vi "TalonFXCommandPosition.vi"(0 "Device Reference (in)":T2, 5 "Output Mode":T1(ring), 7 "Control Mode":enum16{"Safety", "Travelling", "Positioning"}(ring), 9 "Position (counts) or Testing Power":dbl, 11 "Error (in)":errorcluster, 12 "Feed Forward Power [-1, 1]":dbl) -> ()   [LabVIEW 2020]
doc: "Wrapper for commanding the postion of a Talon SRX motor controller. Supports PID, Motion Magic, and a safety interlock. Also supports the standard actuator testing interface and and the only sending new values on change."
uses:
  <vilib>/Rock Robotics/WPI/MotorControl/WPI_MotorControlDeviceRef.ctl
  <vilib>/Rock Robotics/WPI/MotorControl/WPI_MotorControlType.ctl
  <vilib>/Rock Robotics/SystemInterfaces/DIO/FPGA_DIOPWMChannel.ctl
  <vilib>/Rock Robotics/WPI/PWM/WPI_PWMDeadband.ctl
  <vilib>/Rock Robotics/SystemInterfaces/DIO/FPGA_DIOChannel.ctl
  <vilib>/Rock Robotics/WPI/ThirdParty/Phoenix-LabVIEW/Motor Controller/Controls/CTRE_Phoenix_MotorControl_ControlMode.ctl
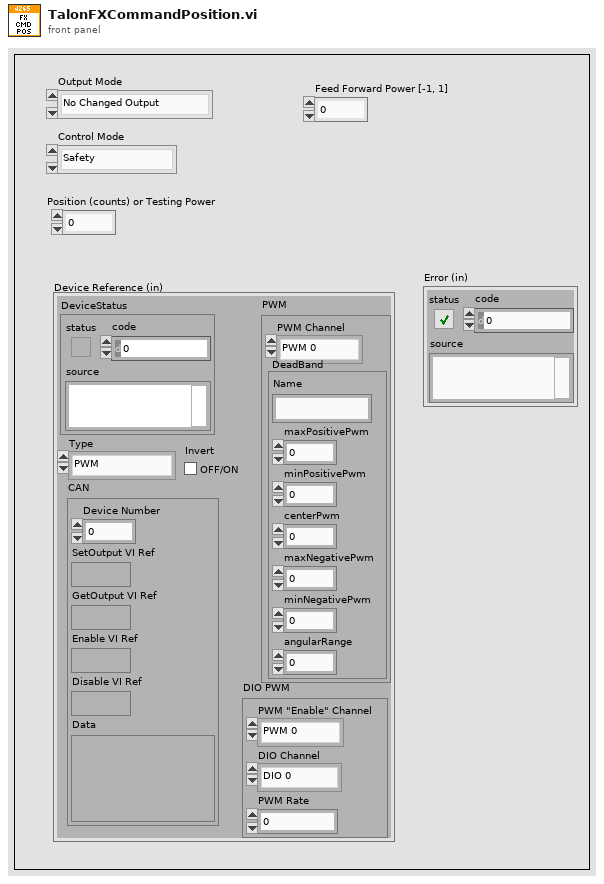
[diagram p1: front panel]
types:
  T1 = enum16{"No Changed Output", "New Normal Output", "New Testing Output"}
  T2 = typedef "WPI_MotorControlDeviceRef.ctl" = cluster{"DeviceStatus":errorcluster, "Type":T3, "PWM":cluster{"PWM Channel":T4, "DeadBand":T5}, "CAN":cluster{"Device Number":u8, "SetOutput VI Ref":variant, "GetOutput VI Ref":variant, "Enable VI Ref":variant, "Disable VI Ref":variant, "Data":variant}, "Invert":bool, "DIO PWM":cluster{"PWM \"Enable\" Channel":T4, "DIOChannel":T6, "PWM Rate":dbl}}
  T3 = typedef "WPI_MotorControlType.ctl" = enum16{"PWM", "CAN", "DIO PWM"}
  T4 = typedef "FPGA_DIOPWMChannel.ctl" = enum8{"PWM 0", "PWM 1", "PWM 2", "PWM 3", "PWM 4", "PWM 5", "PWM 6", "PWM 7", "PWM 8", "PWM 9", "PWM MXP 0", "PWM MXP 1", "PWM MXP 2", "PWM MXP 3", "PWM MXP 4", "PWM MXP 5", "PWM MXP 6", "PWM MXP 7", "PWM MXP 8", "PWM MXP 9", "Invalid"}
  T5 = typedef "WPI_PWMDeadband.ctl" = cluster{"Name":string, "maxPositivePwm":i32, "minPositivePwm":i32, "centerPwm":i32, "maxNegativePwm":i32, "minNegativePwm":i32, "angularRange":u16}
  T6 = typedef "FPGA_DIOChannel.ctl" = enum8{"DIO 0", "DIO 1", "DIO 2", "DIO 3", "DIO 4", "DIO 5", "DIO 6", "DIO 7", "DIO 8", "DIO 9", "DIO MXP 0", "DIO MXP 1", "DIO MXP 2", "DIO MXP 3", "DIO MXP 4", "DIO MXP 5", "DIO MXP 6", "DIO MXP 7", "DIO MXP 8", "DIO MXP 9", "DIO MXP 10", "DIO MXP 11", "DIO MXP 12", "DIO MXP 13", "DIO MXP 14", "DIO MXP 15", "SPI Port CS1", "SPI Port CS2", "SPI Port CS3", "SPI Port MISO", "SPI Port MOSI", "Invalid"}
  T7 = enum16{"DemandType_Neutral", "DemandType_AuxPID", "DemandType_ArbitraryFeedForward"}
  T8 = typedef "CTRE_Phoenix_MotorControl_ControlMode.ctl" = u16
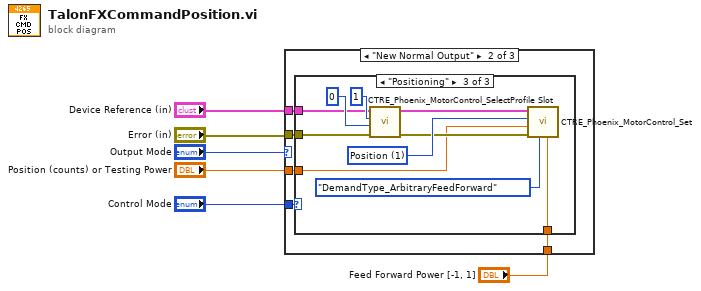
[diagram p0: block diagram]
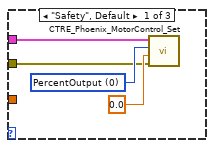
[diagram p3: hidden frame]
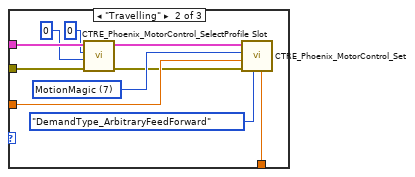
[diagram p4: hidden frame]
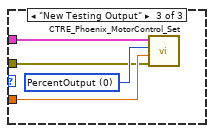
[diagram p5: hidden frame]
diagram:
  n1 = case shown="\"New Normal Output\"" "Output Mode" {
    tunnel: "Position (counts) or Testing Power" -> [_ w10 w38]
    tunnel: "Device Reference (in)" -> [_ w9 w39]
    tunnel: "Feed Forward Power [-1, 1]" -> [_ w11 _]
    tunnel: "Control Mode" -> [_ w8 _]
    tunnel: "Error (in)" -> [_ w7 w36]
    frame "No Changed Output", Default {
    }
    frame "New Normal Output" {
      n2 = case shown="\"Positioning\"" w8 {
        tunnel: w9 -> [w15 w21 w29]
        tunnel: w10 -> [_ w24 w27]
        tunnel: w11 -> [_ w22 w26]
        tunnel: w7 -> [w12 w16 w28]
        frame "Safety", Default {
          w14 = T8 0 items=["PercentOutput"=0, "Position"=1, "Velocity"=2, "Current"=3, "Follower"=5, "MotionProfile"=6, "MotionMagic"=7, "MotionProfileArc"=10, "Disabled"=15] ("Control Mode")
          n3 = call <vilib>:"CTRE_Phoenix_MotorControl_Set.vi"("error in (no error)"=w12, "Output"=0.0, "Control Mode"=w14, "PhoenixMotorControlDevRef"=w15) -> ()  [unwired: 6 in, 2 out]
        }
        frame "Travelling" {
          w25 = T8 7 items=["PercentOutput"=0, "Position"=1, "Velocity"=2, "Current"=3, "Follower"=5, "MotionProfile"=6, "MotionMagic"=7, "MotionProfileArc"=10, "Disabled"=15] ("Control Mode")
          n4 = call <vilib>:"CTRE_Phoenix_MotorControl_SelectProfile Slot.vi"("error in (no error)"=w16, "pidLoopIdx"=0, "slotIdx"=0, "PhoenixMotorControlDevRef"=w21) -> ("error out"=w17:errorcluster, "PhoenixMotorControlDevRef"=w20:T2)  [unwired: 6 in]
          n5 = call <vilib>:"CTRE_Phoenix_MotorControl_Set.vi"("Demand1"=w22, "DemandType"=T7."DemandType_ArbitraryFeedForward", "error in (no error)"=w17, "Output"=w24, "Control Mode"=w25, "PhoenixMotorControlDevRef"=w20) -> ()  [unwired: 4 in, 2 out]
        }
        frame "Positioning" {
          w35 = T8 1 items=["PercentOutput"=0, "Position"=1, "Velocity"=2, "Current"=3, "Follower"=5, "MotionProfile"=6, "MotionMagic"=7, "MotionProfileArc"=10, "Disabled"=15] ("Control Mode")
          n6 = call <vilib>:"CTRE_Phoenix_MotorControl_SelectProfile Slot.vi"("error in (no error)"=w28, "pidLoopIdx"=0, "slotIdx"=1, "PhoenixMotorControlDevRef"=w29) -> ("error out"=w30:errorcluster, "PhoenixMotorControlDevRef"=w33:T2)  [unwired: 6 in]
          n7 = call <vilib>:"CTRE_Phoenix_MotorControl_Set.vi"("Demand1"=w26, "DemandType"=T7."DemandType_ArbitraryFeedForward", "error in (no error)"=w30, "Output"=w27, "Control Mode"=w35, "PhoenixMotorControlDevRef"=w33) -> ()  [unwired: 4 in, 2 out]
        }
      }
    }
    frame "New Testing Output" {
      w37 = T8 0 items=["PercentOutput"=0, "Position"=1, "Velocity"=2, "Current"=3, "Follower"=5, "MotionProfile"=6, "MotionMagic"=7, "MotionProfileArc"=10, "Disabled"=15] ("Control Mode")
      n8 = call <vilib>:"CTRE_Phoenix_MotorControl_Set.vi"("error in (no error)"=w36, "Output"=w38, "Control Mode"=w37, "PhoenixMotorControlDevRef"=w39) -> ()  [unwired: 6 in, 2 out]
    }
  }
